vi "Vision Processing.vi"(8 "error in (no error)":errorcluster, 11 "Image Size":T1=enum."320x240") -> ()   [LabVIEW 2016]
uses:
  Vision Support Code/Camera Types.ctl
  <vilib>/Rock Robotics/WPI/Camera/WPI_CameraImageSize.ctl
  <vilib>/Rock Robotics/WPI/Camera/WPI_CameraWhite Balance Values.ctl
  <vilib>/Rock Robotics/WPI/Camera/WPI_CameraExposure Values.ctl
  <vilib>/Rock Robotics/WPI/Camera/WPI_CameraFrameRate.ctl
  CameraEnum.ctl
  Robot Global Data.vi
  <vilib>/Rock Robotics/Network Tables/NT Read Number.vi
  <vilib>/Rock Robotics/Network Tables/NT Write Number.vi
  <vilib>/vision/NI_Vision_Development_Module.lvlib
panel:
  in  "Use local LED color":bool
  out "loop ms":u32
  out "Calibration error":errorcluster
  in  "Display Original":bool
  in  "Display Mask":bool
  in  "Line Border":cluster{"Top":dbl, "Bottom":dbl}={"Top"=6.0, "Bottom"=1.0}
  in  "Use Calibration":bool
  out "Instructions:":string="Use Source to load image files from a directory, or use a USB or IP camera connected to your laptop. Use Camera Settings 1 and 2 to achieve a dark image with bright and colorful stripes.\nLED Color can encoded as HSL or related color modes. Calibrate to the same color as the strips being reflected to the camera.\nClick and draw a line in Original Image to auto-calibrate the LED Color. You may want to widen and tweak Sat and Val by hand.\nThe Annotate button affects drawing a rectangle around the stripes and labeling it with a distance in ft. Distance relies on knowing the Camera Type and lens calibration (it looks up the lens view angle).\n\nAdjust Score Cutoff to make the code more or less picky. If the color is not very unique, you may need to increase the number of particles considered. The diagram uses a Size Limit to ignore colored things that are too small. You may need to adjust it if you are targetting from far away.\n\nResults give you the distance to the target, the center and box in a normalized (-1 to 1) and pixel coordinates.\n\nBe sure to read about setting camera exposure and brightness to help simplify your image and acquire color saturated images.\n\nThere are lots of comments on the diagram to explain the code."
  in  "Color Mode":u16(ring)=3 items=["RGB", "HSL", "HSV", "HSI"]
  in  "Particles":dbl=5.0
  in  "Score Cutoff %":dbl=70.0
  in  "Camera Type":T2=enum."MS HD3000 square"
  out "Results":T3 {"Score" format="%#_3g"; "Pixels"."Rectangle"."Numeric 5" format="%#_3g"; "Pixels"."Rectangle"."Numeric 3" format="%#_3g"; "Pixels"."Rectangle"."Numeric 2" format="%#_3g"; "Pixels"."Rectangle"."Numeric" format="%#_3g"; "Normalized"."Rectangle"."Numeric 5" format="%#_2g"; "Normalized"."Rectangle"."Numeric 3" format="%#_2g"; "Normalized"."Rectangle"."Numeric 2" format="%#_2g"; "Normalized"."Rectangle"."Numeric" format="%#_2g"; "Normalized"."Center"."?" format="%#_3g"; "Normalized"."Center"."?" format="%#_3g"; "Distance (ft)" format="%#_3g"}
  out "Qualified Particles":i32
  in  "LED Color":T4={"Hue"={107.81818389892578, 139.81818389892578}, "Sat"={176.07142857142858, 255.0}, "Val"={40.53571428571429, 255.0}} {"Hue" scale=0.0..255.0 scale format="%#_3g"}
  out "Mask":T5(plugin-control)
  out "Original Image":T5(plugin-control)
  # "Legend:\n    Rectangle\n       Green - Good target, distance ft\n       Red - Bad target\n    Orange Text - Score in %"
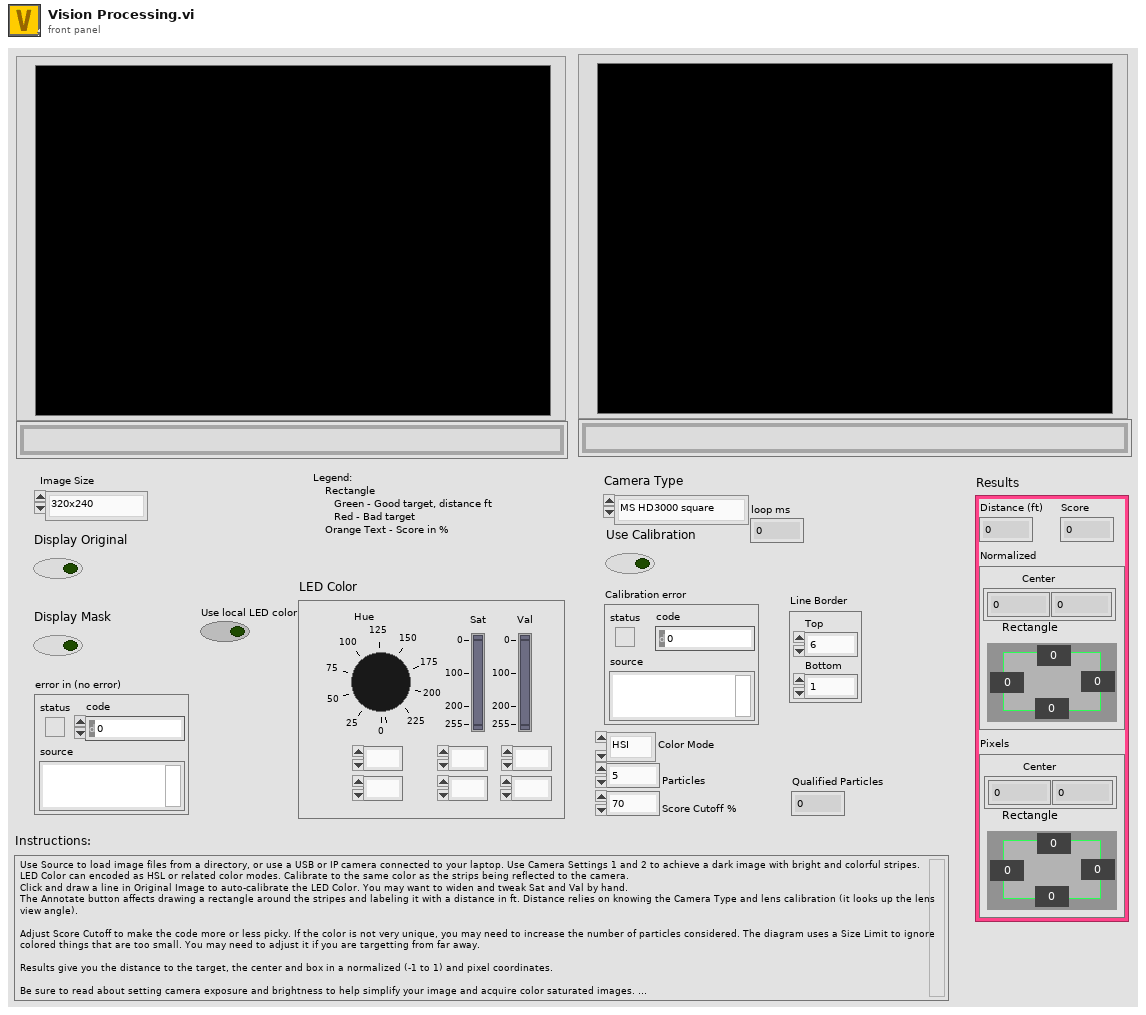
[diagram p1: front panel]
types:
  T1 = typedef "WPI_CameraImageSize.ctl" = enum16{"640x480", "320x240", "160x120", "Custom"}
  T2 = typedef "Camera Types.ctl" = enum16{"206", "1011", "1013", "MS HD3000 square", "MS HD3000 640x480"}
  T3 = cluster{"Distance (ft)":dbl, "Score":dbl, "Normalized":cluster{"Center":cluster{dbl, dbl}, "Rectangle":cluster{"Numeric":dbl, "Numeric 2":dbl, "Numeric 3":dbl, "Numeric 5":dbl}}, "Pixels":cluster{"Center":cluster{dbl, dbl}, "Rectangle":cluster{"Numeric":dbl, "Numeric 2":dbl, "Numeric 3":dbl, "Numeric 5":dbl}}}
  T4 = cluster{"Hue":cluster{dbl, dbl}, "Sat":cluster{dbl, dbl}, "Val":cluster{dbl, dbl}}
  T5 = typedef "IMAQ Image.ctl" = refnum<image>
  T6 = typedef "Image Type" = u32
  T7 = typedef "WPI_CameraFrameRate.ctl" = u32
  T8 = typedef "WPI_CameraExposure Values.ctl" = enum16{"Auto", "Flicker-free 50 Hz", "Flicker-free 60 Hz", "Hold current", "Custom"}
  T9 = typedef "WPI_CameraWhite Balance Values.ctl" = enum16{"Auto", "Fixed indoor", "Fixed outdoor 1", "Fixed outdoor 2", "Fixed fluorescent 1", "Fixed fluorescent 2", "Hold current", "Custom"}
  T10 = typedef "Particle Parameters" = i32
  T11 = typedef "WPI_CameraDevRef.ctl" = cluster{"Camera Address":string, "CameraStatus":errorcluster}
  T12 = typedef "CameraEnum.ctl" = enum16{"Front", "Back"}
  T13 = cluster{cluster{"Hue Min":dbl, "Hue Max":dbl}, cluster{"Sat Min":dbl, "Sat Max":dbl}, cluster{"Val Min":dbl, "Val Max":dbl}}
  T14 = cluster{"Left":dbl, "Top":dbl, "Right":dbl, "Bottom":dbl}
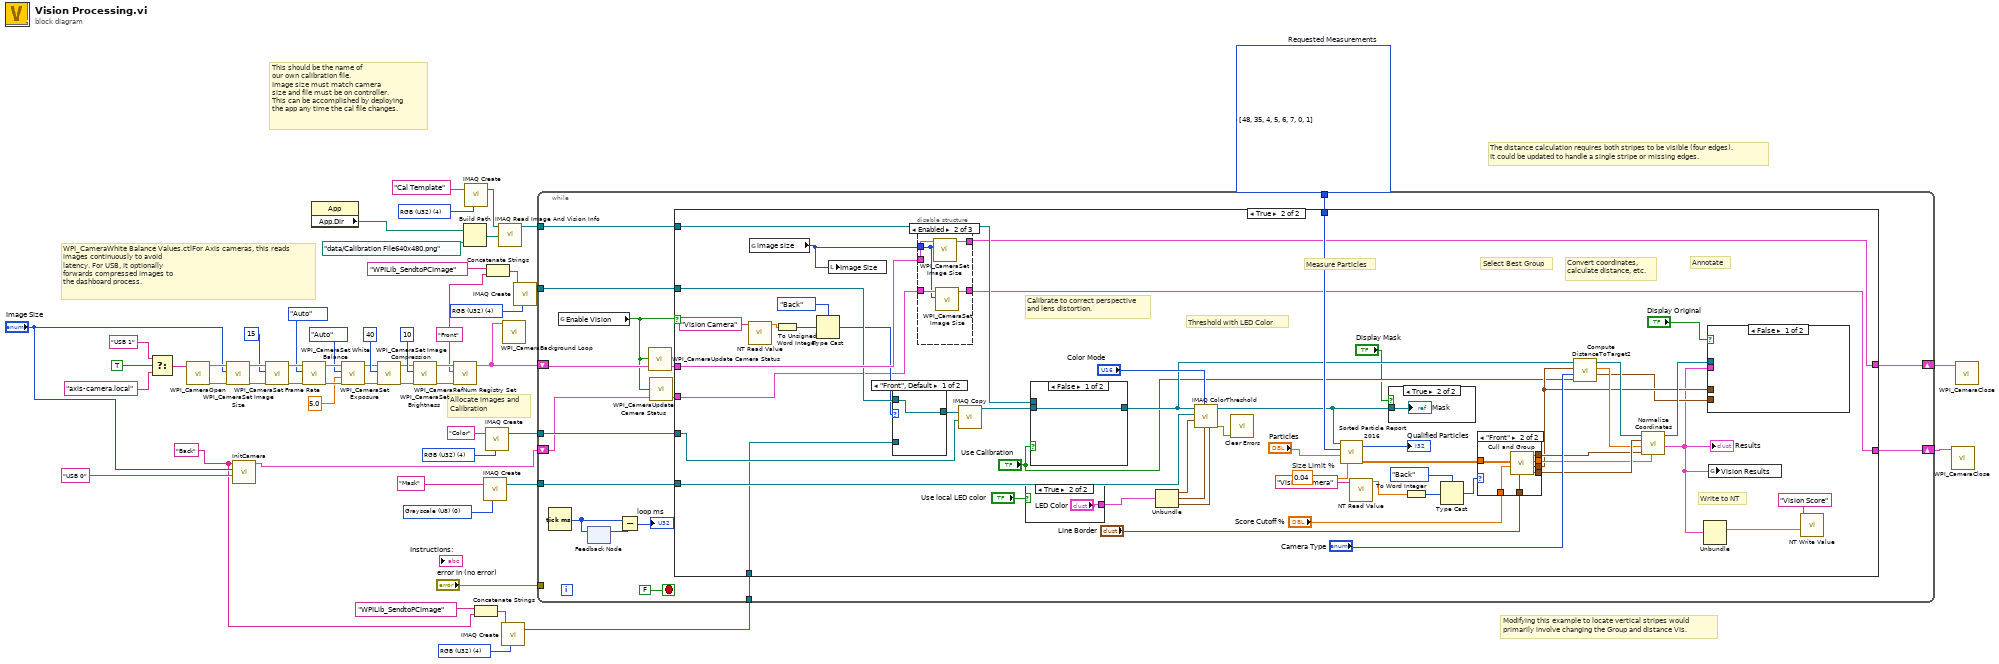
[diagram p0: block diagram]
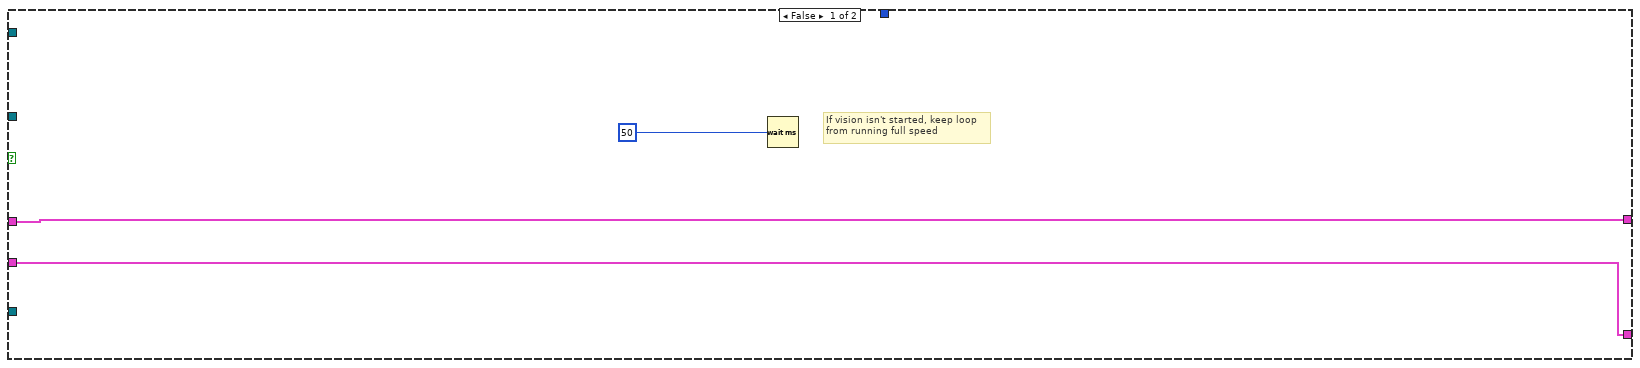
[diagram p2: hidden frame]
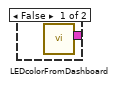
[diagram p3: hidden frame]
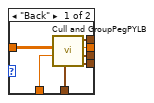
[diagram p4: hidden frame]
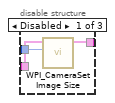
[diagram p5: hidden frame]
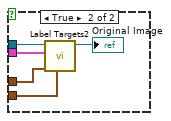
[diagram p8: hidden frame]
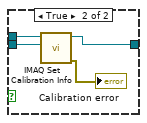
[diagram p10: hidden frame]
diagram:
  w3 = T6 4 items=["Grayscale (U8)", "Grayscale (I16)", "Grayscale (SGL)", "Complex (CSG)", "RGB (U32)", "HSL (U32)", "RGB (U64)", "Grayscale (U16)"] ("Image Type")
  w10 = T6 4 items=["Grayscale (U8)", "Grayscale (I16)", "Grayscale (SGL)", "Complex (CSG)", "RGB (U32)", "HSL (U32)", "RGB (U64)", "Grayscale (U16)"] ("Image Type")
  w6 = "Back" ("refnum name")
  w2 = "Front" ("refnum name")
  w48 = T6 4 items=["Grayscale (U8)", "Grayscale (I16)", "Grayscale (SGL)", "Complex (CSG)", "RGB (U32)", "HSL (U32)", "RGB (U64)", "Grayscale (U16)"] ("Image Type")
  w50 = T10[] [48, 35, 4, 5, 6, 7, 0, 1] items=["Center of Mass X", "Center of Mass Y", "First Pixel X", "First Pixel Y", "Bounding Rect Left", "Bounding Rect Top", "Bounding Rect Right", "Bounding Rect Bottom", "Max Feret Diameter Start X", "Max Feret Diameter Start Y", "Max Feret Diameter End X", "Max Feret Diameter End Y", "Max Horiz. Segment Length Left", "Max Horiz. Segment Length Right", "Max Horiz. Segment Length Row", "-", "Bounding Rect Width", "Bounding Rect Height", "Bounding Rect Diagonal", "Perimeter", "Convex Hull Perimeter", "Holes' Perimeter", "Max Feret Diameter", "Equivalent Ellipse Major Axis", "Equivalent Ellipse Minor Axis", "Equivalent Ellipse Minor Axis (Feret)", "Equivalent Rect Long Side", "Equivalent Rect Short Side", "Equivalent Rect Diagonal", "Equivalent Rect Short Side (Feret)", "Average Horiz. Segment Length", "Average Vert. Segment Length", "Hydraulic Radius", "Waddel Disk Diameter", "-", "Area", "Holes' Area", "Particle & Holes' Area", "Convex Hull Area", "Image Area", "-", "Number of Holes", "Number of Horiz. Segments", "Number of Vert. Segments", "-", "Orientation", "Max Feret Diameter Orientation", "-", "% Area/Image Area", "% Area/(Particle & Holes' Area)", "Ratio of Equivalent Ellipse Axes", "Ratio of Equivalent Rect Sides", "-", "Elongation Factor", "Compactness Factor", "Heywood Circularity Factor", "Type Factor", "-", "Sum X", "Sum Y", "Sum XX", "Sum XY", "Sum YY", "Sum XXX", "Sum XXY", "Sum XYY", "Sum YYY", "-", "Moment of Inertia XX", "Moment of Inertia XY", "Moment of Inertia YY", "Moment of Inertia XXX", "Moment of Inertia XXY", "Moment of Inertia XYY", "Moment of Inertia YYY", "Norm. Moment of Inertia XX", "Norm. Moment of Inertia XY", "Norm. Moment of Inertia YY", "Norm. Moment of Inertia XXX", "Norm. Moment of Inertia XXY", "Norm. Moment of Inertia XYY", "Norm. Moment of Inertia YYY", "Hu Moment 1", "Hu Moment 2", "Hu Moment 3", "Hu Moment 4", "Hu Moment 5", "Hu Moment 6", "Hu Moment 7"]  # Requested Measurements
  w53 = T6 0 items=["Grayscale (U8)", "Grayscale (I16)", "Grayscale (SGL)", "Complex (CSG)", "RGB (U32)", "HSL (U32)", "RGB (U64)", "Grayscale (U16)"] ("Image Type")
  w54 = T6 4 items=["Grayscale (U8)", "Grayscale (I16)", "Grayscale (SGL)", "Complex (CSG)", "RGB (U32)", "HSL (U32)", "RGB (U64)", "Grayscale (U16)"] ("Image Type")
  # "This should be the name of \nour own calibration file.\nImage size must match camera\nsize and file must be on controller.\nThis can be accomplished by deploying\nthe app any time the cal file changes."
  # "WPI_CameraWhite Balance Values.ctlFor Axis cameras, this reads\nimages continuously to avoid\nlatency. For USB, it optionally\nforwards compressed images to\nthe dashboard process."
  # "Modifying this example to locate vertical stripes would\nprimarily involve changing the Group and distance VIs."
  # "The distance calculation requires both stripes to be visible (four edges).\nIt could be updated to handle a single stripe or missing edges."
  # "Allocate images and\nCalibration"
  n1 = Select(t="USB 1" ("format string"), s=TRUE ("dot notation? (F)"), f="axis-camera.local" ("format string")) -> (s? t:f=w20:string)
  n2 = call <vilib>:"WPI_CameraOpen.vi"("Camera Address"=w20) -> ("error out"=w32:errorcluster, "CameraDevRef"=w33:T11)  [unwired: 1 in, 8 out]
  n3 = call <vilib>:"WPI_CameraSet Image Size.vi"("error in (no error)"=w32, "Image Size"="Image Size", "CameraDevRef"=w33) -> ("error out"=w31:errorcluster, "CameraDevRef Out"=w34:T11)  [unwired: 1 in, 6 out]
  n4 = call "InitCamera.vi"("format string"="USB 0", "Image Size"="Image Size", "refnum name"=w6) -> ("CameraDevRef"=w12:T11)  [unwired: 8 in]
  n5 = call <vilib>:"WPI_CameraSet Frame Rate.vi"("error in (no error)"=w31, "Frame Rate (fps)"=T7 15, "CameraDevRef"=w34) -> ("error out"=w30:errorcluster, "CameraDevRef Out"=w36:T11)  [unwired: 7 out]
  n6 = call <vilib>:"WPI_CameraSet White Balance.vi"("error in (no error)"=w30, "White Balance"=WPI_CameraWhite_Balance_Values."Auto", "CameraDevRef"=w36) -> ("error out"=w29:errorcluster, "CameraDevRef Out"=w35:T11)  [unwired: 1 in, 6 out]
  n7 = property class="App"() -> ("App.Dir"=w15:path)  [unwired: 2 in, 2 out]
  n8 = call <vilib>:"WPI_CameraSet Exposure.vi"("error in (no error)"=w29, "Exposure (%)"=5.0, "Exposure"=WPI_CameraExposure_Values."Auto", "CameraDevRef"=w35) -> ("error out"=w28:errorcluster, "CameraDevRef Out"=w38:T11)  [unwired: 6 out]
  n9 = call <vilib>:"WPI_CameraSet Image Compression.vi"("error in (no error)"=w28, "Compression"=40, "CameraDevRef"=w38) -> ("error out"=w27:errorcluster, "CameraDevRef Out"=w37:T11)  [unwired: 7 out]
  n10 = call <vilib>:"WPI_CameraSet Brightness.vi"("error in (no error)"=w27, "Brightness"=10, "CameraDevRef"=w37) -> ("error out"=w26:errorcluster, "CameraDevRef Out"=w42:T11)  [unwired: 7 out]
  n11 = call <vilib>:"WPI_CameraRefNum Registry Set.vi"("error in (no error)"=w26, "refnum name"=w2, "CameraDevRef"=w42) -> ("CameraDevRef"=w19:T11)  [unwired: 1 in, 7 out]
  n12 = Build Path(base path=w15, name or relative path=path "data/Calibration File640x480.png" ("Folder Location")) -> (appended path=w44:path)
  n13 = call "IMAQ Create"("Image Name"="Cal Template", "Image Type"=w48) -> ("New Image"=w46:T5)  [unwired: 2 in, 2 out]
  n14 = Concatenate Strings("WPILib_SendtoPCImage", w6) -> (w9:string)
  n15 = call "IMAQ Create"("Image Name"="Mask", "Image Type"=w53) -> ("New Image"=w51:T5)  [unwired: 2 in, 2 out]
  n16 = call "IMAQ Create"("Image Name"="Color", "Image Type"=w54) -> ("New Image"=w49:T5)  [unwired: 2 in, 2 out]
  n17 = Concatenate Strings("WPILib_SendtoPCImage", w2) -> (w4:string)
  n18 = call "IMAQ Read Image And Vision Info"("File Path"=w44, "Image"=w46) -> ("Image Out"=w45:T5)  [unwired: 7 in, 2 out]
  n19 = call "IMAQ Create"("Image Name"=w9, "Image Type"=w10) -> ("New Image"=w7:T5)  [unwired: 2 in, 2 out]
  n20 = call <vilib>:"WPI_CameraBackground Loop.vi"("CameraDevRef"=w19) -> ()  [unwired: 11 in]
  n21 = call "IMAQ Create"("Image Name"=w4, "Image Type"=w3) -> ("New Image"=w1:T5)  [unwired: 2 in, 2 out]
  n22 = while {
    tunnel: w49 -> [w68]
    tunnel: w51 -> [w71]
    tunnel: w50 -> [w70]
    tunnel: w45 -> [w69]
    shift-right: [w67] -> w18
    shift-left: w19 -> [w66]
    tunnel: "error in (no error)" -> [_]
    shift-right: [w61] -> w13
    shift-left: w12 -> [w59]
    tunnel: w7 -> [w57]
    tunnel: w1 -> [w56]
    stop <- FALSE stop-if-true
    n23 = Tick Count (ms)() -> (millisecond timer value=w63:u32)
    n24 = global read "Robot Global Data.vi" "Enable Vision"() -> (w60:bool)
    n25 = feedback-in #1(w63) -> ()
    n26 = feedback #1() -> (w64:u32)  [unwired: 1 in]
    n27 = Subtract(x=w63, y=w64) -> (x-y=→"loop ms":u32)
    n28 = call <vilib>:"WPI_CameraUpdate Camera Status.vi"("CameraDevRef In"=w66, "Enable Vision"=w60) -> ("CameraDevRef Out"=w65:T11)  [unwired: 3 in]
    n29 = call <vilib>:"WPI_CameraUpdate Camera Status.vi"("CameraDevRef In"=w59, "Enable Vision"=w60) -> ("CameraDevRef Out"=w58:T11)  [unwired: 3 in]
    n30 = case shown="True" w60 {
      tunnel: w71 -> [_ w128]
      tunnel: w70 -> [_ w124]
      tunnel: w69 -> [_ w104]
      tunnel: w65 -> [w75 w92]
      tunnel: w68 -> [_ w101]
      tunnel: [w75 w97] -> w67
      tunnel: [w73 w82] -> w61
      tunnel: w58 -> [w73 w83]
      tunnel: w57 -> [_ w89]
      tunnel: w56 -> [_ w88]
      frame False {
        # "If vision isn't started, keep loop\nfrom running full speed"
        n31 = Wait (ms)(milliseconds to wait=u32 50) -> ()  [unwired: 1 out]
      }
      frame True {
        w122 = 0.04  # Size Limit %
        # "Write to NT"
        # "Calibrate to correct perspective\nand lens distortion."
        # "Measure Particles"
        # "Convert coordinates,\ncalculate distance, etc."
        # "Annotate"
        # "Select Best Group"
        # "Threshold with LED Color"
        n32 = call-poly <vilib>:"NT Read Value.vi"("Name"="Vision Camera") -> ("Numeric"=w86:dbl)  [unwired: 9 in, 1 out]
        n33 = global read "Robot Global Data.vi" "image size"() -> (w96:T1)
        n34 = To Unsigned Word Integer(number=w86) -> (unsigned 16bit integer=w87:u16)
        n35 = Type Cast(type=CameraEnum."Back", x=w87) -> (*(type *) &x=w85:T12)
        n36 = local write "Image Size"(w96) -> ()
        n37 = case shown="\"Front\", Default" w85 {
          tunnel: [w154 w155] -> w90
          tunnel: w89 -> [_ w155]
          tunnel: w88 -> [w154 _]
          frame "Front", Default {
          }
          frame "Back" {
          }
        }
        n38 = disable-structure shown="Enabled" {
          disable-tunnel: [w147 w152 w153] -> w97
          disable-tunnel: w96 -> [w146 w149 _]
          disable-tunnel: w92 -> [w145 w151 w153]
          disable-tunnel: w83 -> [_ w150 _]
          disable-tunnel: [_ w148 _] -> w82
          frame Disabled {
            n39 = call <vilib>:"WPI_CameraSet Image Size.vi"("Image Size"=w146, "CameraDevRef"=w145) -> ("CameraDevRef Out"=w147:T11)  [unwired: 2 in, 7 out]
          }
          frame Enabled {
            n40 = call <vilib>:"WPI_CameraSet Image Size.vi"("Image Size"=w149, "CameraDevRef"=w151) -> ("CameraDevRef Out"=w152:T11)  [unwired: 2 in, 7 out]
            n41 = call <vilib>:"WPI_CameraSet Image Size.vi"("Image Size"=w149, "CameraDevRef"=w150) -> ("CameraDevRef Out"=w148:T11)  [unwired: 2 in, 7 out]
          }
          frame Disabled {
          }
        }
        n42 = call "IMAQ Copy"("Image Dst"=w101, "Image Src"=w90) -> ("Image Dst Out"=w100:T5)  [unwired: 4 in, 1 out]
        n43 = case shown="True" "Use local LED color" {
          tunnel: [w129 "LED Color"] -> w120
          frame False {
            n44 = call "LEDcolorFromDashboard.vi"() -> ("LED color"=w129:T13)  [unwired: 11 in]
          }
          frame True {
          }
        }
        n45 = case shown="False" "Use Calibration" {
          tunnel: [w162 w166] -> w105
          tunnel: w100 -> [w162 w165]
          tunnel: w104 -> [_ w164]
          frame False {
          }
          frame True {
            n46 = call "IMAQ Set Calibration Info"("Image Dst"=w165, "Image Src"=w164) -> ("error out"=→"Calibration error":errorcluster, "Calibrated Image"=w166:T5)  [unwired: 8 in]
          }
        }
        n47 = Unbundle(w120) -> ("Hue"=w127:cluster{"Hue Min":dbl, "Hue Max":dbl}, "Sat"=w126:cluster{"Sat Min":dbl, "Sat Max":dbl}, "Val"=w125:cluster{"Val Min":dbl, "Val Max":dbl})
        n48 = call "IMAQ ColorThreshold"("Blue or Luma or Val or Inten Range"=w125, "Green or Sat Range"=w126, "Color Mode"="Color Mode", "Red or Hue Range"=w127, "Image Dst"=w128, "Image Src"=w105) -> ("error out"=w121:errorcluster, "Image Dst Out"=w117:T5)  [unwired: 4 in]
        n49 = call <vilib>:"Clear Errors.vi"("error in (no error)"=w121) -> ()  [unwired: 5 in, 2 out]
        n50 = call "Sorted Particle Report 2016.vi"("Min Area Size %"=w122, "Particle Count Limit"="Particles", "Pixel Measurements"=w124, "Image in"=w117) -> ("Sorted Data"=w119:dbl[][], "Particles"=→"Qualified Particles":i32)
        n51 = call-poly <vilib>:"NT Read Value.vi"("Name"="Vision Camera") -> ("Numeric"=w80:dbl)  [unwired: 9 in, 1 out]
        n52 = case shown="True" "Display Mask" {
          tunnel: w117 -> [_ w161]
          frame False {
          }
          frame True {
            "Mask" <- w161
          }
        }
        n53 = To Word Integer(number=w80) -> (16bit integer=w79:i16)
        n54 = Type Cast(type=CameraEnum."Back" ("Vision Camera"), x=w79) -> (*(type *) &x=w77:T12)
        n55 = case shown="\"Front\"" w77 {
          tunnel: w119 -> [w137 w144]
          tunnel: "Score Cutoff %" -> [w136 w143]
          tunnel: [w135 w142] -> w115
          tunnel: [w134 w141] -> w111
          tunnel: [w133 w140] -> w110
          tunnel: [w132 w139] -> w107
          tunnel: "Line Border" -> [w131 w138]
          frame "Back" {
            n56 = call "Cull and GroupPegPYLB.vi"("Line Border"=w131, "Score Cutoff"=w136, "Sorted Data"=w137) -> ("Rect"=w135:T14, "Line"=w132:T14, "Score"=w133:dbl, "Center"=w134:cluster{"X":dbl, "Y":dbl})  [unwired: 5 in]
          }
          frame "Front" {
            n57 = call "Cull and Group.vi"("Line Border"=w138, "Score Cutoff"=w143, "Sorted Data"=w144) -> ("Rect"=w142:T14, "Line"=w139:T14, "Score"=w140:dbl, "Center"=w141:cluster{"X":dbl, "Y":dbl})  [unwired: 5 in]
          }
        }
        n58 = call "Compute DistanceToTarget2.vi"("Calibrated"="Use Calibration", "Camera Type"="Camera Type", "Line"=w107, "Image Src"=w105) -> ("Edges"=w106:cluster{"X":sgl, "Y":sgl}[], "Distance (ft)"=w114:dbl, "Image Dst Out"=w113:T5)  [unwired: 5 in]
        n59 = call "Normalize Coordinates.vi"("Score"=w110, "Center"=w111, "Distance"=w114, "Bounding box"=w115, "Image in"=w113) -> ("Results"=w95:T3, "Image out"=w112:T5)  [unwired: 5 in]
        "Results" <- w95
        n60 = Unbundle(w95) -> ("Score"=w94:dbl)  [unwired: 3 out]
        n61 = case shown="False" "Display Original" {
          tunnel: w112 -> [_ w159]
          tunnel: w95 -> [_ w158]
          tunnel: w107 -> [_ w157]
          tunnel: w106 -> [_ w156]
          frame False {
          }
          frame True {
            n62 = call "Label Targets2.vi"("Edges"=w156, "Line"=w157, "Results"=w158, "Image in"=w159) -> ("Image out"=→"Original Image":T5)  [unwired: 7 in]
          }
        }
        n63 = global write "Robot Global Data.vi" "Vision Results"(w95) -> ()
        n64 = call-poly <vilib>:"NT Write Value.vi"("Numeric"=w94, "Name"="Vision Score") -> ()  [unwired: 9 in, 1 out]
      }
    }
  }
  n65 = call <vilib>:"WPI_CameraClose.vi"("CameraDevRef"=w13) -> ()  [unwired: 1 in, 10 out]
  n66 = call <vilib>:"WPI_CameraClose.vi"("CameraDevRef"=w18) -> ()  [unwired: 1 in, 10 out]
